vi "Eagle_FPGA Calc & Check Point.vi"(7 "Calib Values":T1={"X MULT"=-0.024993896484375, "Y MULT"=-0.033294677734375, "X OFFS"=0.0, "Y OFFS"=10.0}, 8 "NoGO Zone":T2, 9 "Center":cluster{"CX":fxp<+,10,10>, "CY":fxp<+,10,10>}, 10 "PX":fxp<+/-,10,11>, 11 "PY":fxp<+/-,10,11>) -> (0 "SCAN ENA":bool, 2 "VY CMD":fxp<+/-,32,17>, 3 "VX CMD":fxp<+/-,32,17>)   [LabVIEW 2015]
uses:
  <vilib>/rvi/interface/RandomDataEmulation/nirviRandomDataMultiElementFPGAFIFO.vi
  <instcachedir>/0/nirviRandomDataMultiElementFPGAFIFO_8F99493546E24284B0D6A8E519C457F7.lvgen/nirviRandomDataMultiElementFPGAFIFO_8F99493546E24284B0D6A8E519C457F7_003.vi
  <vilib>/rvi/interface/RandomDataEmulation/niFpgaRandomDataHandleErrors.vi
  <vilib>/rvi/FXPMathLib/FxpAdd/XNode/nifxpmath_Add.xnode
  <vilib>/rvi/FXPMathLib/FxpMul/XNode/nifxpmath_Multiplier.xnode
  <vilib>/rvi/DataTransferAndStorage/Container/XNode/niFpgaContainer.xnode
  <vilib>/rvi/interface/RandomDataEmulation/nirviRandomDataFpgaMultiElementTemplate.vi
  <vilib>/rvi/FXPMathLib/sim/FxpSim.dll
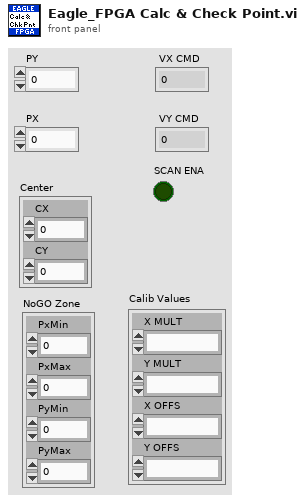
[diagram p1: front panel]
types:
  T1 = cluster{"X MULT":fxp<+/-,20,5>, "Y MULT":fxp<+/-,20,5>, "X OFFS":fxp<+/-,20,5>, "Y OFFS":fxp<+/-,20,5>}
  T2 = cluster{"PxMin":fxp<+,10,10>, "PxMax":fxp<+,10,10>, "PyMin":fxp<+,10,10>, "PyMax":fxp<+,10,10>}
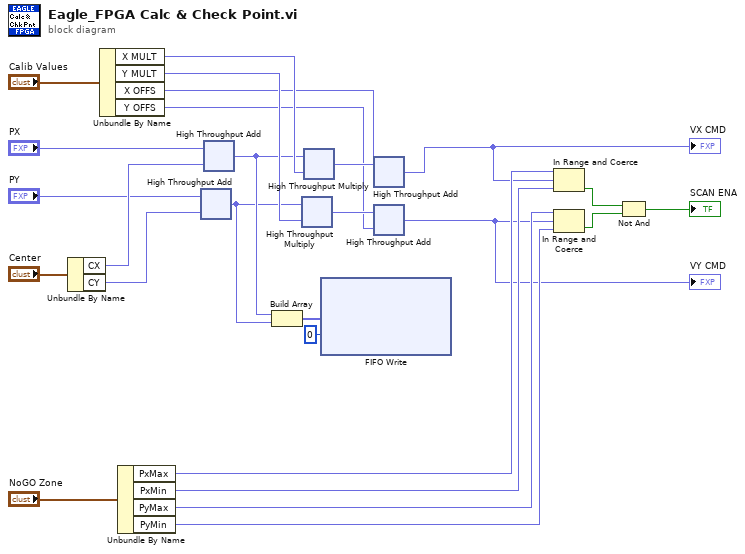
[diagram p0: block diagram]
diagram:
  n1 = Unbundle By Name("Center") -> ("CX"=w23:fxp<+,10,10>, "CY"=w14:fxp<+,10,10>)
  n2 = Unbundle By Name("Calib Values") -> ("X MULT"=w12:fxp<+/-,20,5>, "Y MULT"=w11:fxp<+/-,20,5>, "X OFFS"=w10:fxp<+/-,20,5>, "Y OFFS"=w9:fxp<+/-,20,5>)
  n3 = Unbundle By Name("NoGO Zone") -> ("PxMax"=w21:fxp<+,10,10>, "PxMin"=w20:fxp<+,10,10>, "PyMax"=w19:fxp<+,10,10>, "PyMin"=w18:fxp<+,10,10>)
  n4 = xnode ("High Throughput Add")("x"="PY", "y"=w14) -> ("x+y"=w3:fxp<+/-,12,12>)
  n5 = xnode ("High Throughput Add")("x"="PX", "y"=w23) -> ("x+y"=w4:fxp<+/-,12,12>)
  n6 = Build Array(w4, w3) -> (w2:fxp<+/-,12,12>[])
  n7 = xnode ("High Throughput Multiply")("x"=w3, "y"=w11) -> ("x*y"=w26:fxp<+/-,32,17>)
  n8 = xnode ("High Throughput Multiply")("x"=w4, "y"=w12) -> ("x*y"=w25:fxp<+/-,32,17>)
  n9 = xnode ("FIFO Write")("Element"=w2, "Timeout"=0) -> ()  [unwired: 1 in, 2 out]
  n10 = xnode ("High Throughput Add")("x"=w25, "y"=w10) -> ("x+y"=w8:fxp<+/-,33,18>)
  "VX CMD" <- w8
  n11 = xnode ("High Throughput Add")("x"=w26, "y"=w9) -> ("x+y"=w7:fxp<+/-,33,18>)
  "VY CMD" <- w7
  n12 = In Range and Coerce(upper limit=w21, x=w8, lower limit=w20) -> (In Range?=w17:bool)  [unwired: 1 out]
  n13 = In Range and Coerce(upper limit=w19, x=w7, lower limit=w18) -> (In Range?=w16:bool)  [unwired: 1 out]
  n14 = Not And(1:w16, 2:w17) -> (0:→"SCAN ENA":bool)
